vi "TheCoordinateColor_171213.vi"(6 "InputSegments":bool[](array[boolean]), 8 "X":i32, 9 "Y":i32, 10 "InputSegments(s)":dbl[](array[numeric])) -> (1 "MATCH index":i32, 2 "Outputsegments":bool[](array[boolean]), 3 "OutputSegmens(s)":dbl[](array[numeric]))   [LabVIEW 2016]
uses:
  Globaltracker.vi
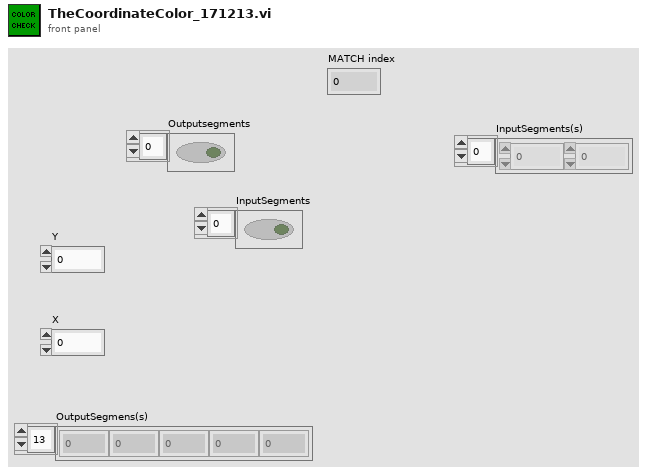
[diagram p1: front panel]
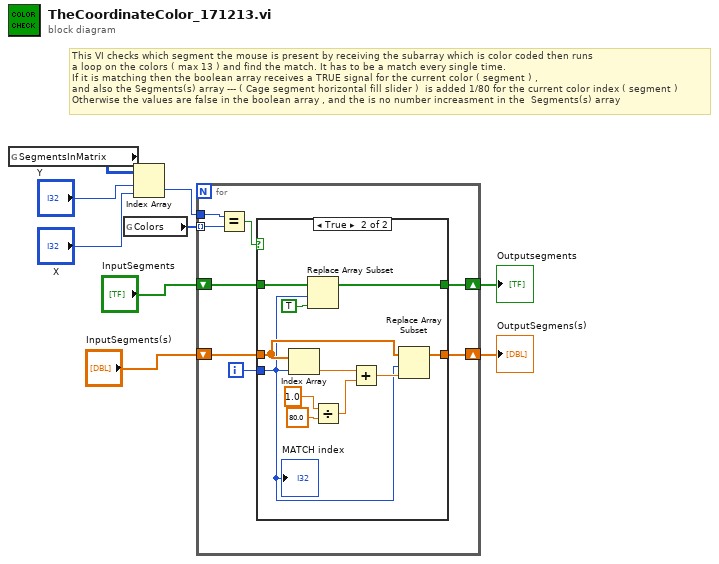
[diagram p0: block diagram]
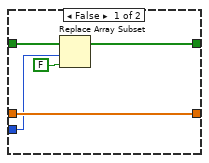
[diagram p2: hidden frame]
diagram:
  # "This VI checks which segment the mouse is present by receiving the subarray which is color coded then runs\na loop on the colors ( max 13 ) and find the match. It has to be a match every single time. \nIf it is matching then the boolean array receives a TRUE signal for the current color ( segment ) , \nand also the Segments(s) array --- ( Cage segment horizontal fill slider )  is added 1/80 for the current color index ( segment ) \nOtherwise the values are false in the boolean array , and the is no number increasment in the  Segments(s) array"
  n1 = global read "Globaltracker.vi" "SegmentsInMatrix"() -> (w4:u32[][])
  n2 = global read "Globaltracker.vi" "Colors"() -> (w5:u32[])
  n3 = Index Array(array=w4, index (row)="Y", index (col)="X") -> (element=w3:u32)
  n4 = for {
    tunnel: w5 -> [w17] mode=indexing
    tunnel: w3 -> [w16]
    shift-right: [w12] -> w7
    shift-left: "InputSegments(s)" -> [w10]
    shift-right: [w11] -> w9
    shift-left: "InputSegments" -> [w13]
    i -> [w14]
    n5 = Equal?(x=w16, y=w17) -> (x = y?=w15:bool)
    n6 = case shown="True" w15 {
      tunnel: w14 -> [w18 w23]
      tunnel: [w22 w29] -> w12
      tunnel: w10 -> [w22 w33]
      tunnel: w13 -> [w21 w32]
      tunnel: [w20 w30] -> w11
      frame False {
        n7 = Replace Array Subset(array=w21, new element=FALSE ("new element/subarray"), index=w18) -> (w20:bool[])
      }
      frame True {
        n8 = Index Array(array=w33, index=w23) -> (element=w28:dbl)
        n9 = Replace Array Subset(array=w32, new element=TRUE ("new element/subarray"), index=w23) -> (w30:bool[])
        n10 = Divide(x=1.0, y=80.0) -> (x/y=w27:dbl)
        n11 = Add(x=w28, y=w27) -> (x+y=w24:dbl)
        n12 = Replace Array Subset(array=w33, new element=w24, index=w23) -> (w29:dbl[])
        "MATCH index" <- w23
      }
    }
  }
  "Outputsegments" <- w9
  "OutputSegmens(s)" <- w7
